vi "Find Repeating Monoclinic GB.vi"(6 "Min Wedge Thickness (A)":dbl=5.0, 8 "Tolerance (A)":dbl=0.5, 9 "Slab Y":dbl=6.0, 10 "Slab X":dbl=6.0, 11 "Supercell Structure":T2={"Structure Name"="CdTe Expanded to Box", "Lattice vector a"=[19.0, 0.0, 0.0], "Lattice vector b"=[0.0, 90.0, 0.0], "Lattice vector c"=[0.0, 0.0, 19.98181818181818], "Atoms Array"=[{"Atom Name"="Cd", "Positions (Direct)"=array501x3[1503 elements], "Positions (Cartesian)"=array501x3[1503 elements]}, {"Atom Name"="Te", "Positions (Direct)"=array504x3[1512 elements], "Positions (Cartesian)"=array504x3[1512 elements]}], "# of atoms"=1005} {"Atoms Array"."Positions (Cartesian)" format="%#_4f"; "Atoms Array"."Positions (Direct)" format="%#_4f"}) -> (1 "Area":dbl, 2 "New Lattice Vector b":dbl[](array[numeric]), 3 "New Lattice Vector a":dbl[](array[numeric]))   [LabVIEW 2010]
panel:
  out "Array 3":dbl[][](array[numeric])
  out "proj":dbl
  out "Possibles from atom 1":dbl[][](array[numeric])
  out "Array 2":dbl[][](array[numeric])
  out "sorted array 2":T1(array[cluster])
  out "All Possible Lattice Vectors":dbl[][](array[numeric]) format="%#_4g"
  out "Slab subset 2":T3(array[cluster])=[{"Atom Name"="Cd", "Positions (Cartesian)"=[[0.0, 4.670554880088597, 0.7469022070093141], [0.0, 0.0, 1.0119047619047619], [0.0, 4.935557434984045, 5.417457087097911], [0.0, 0.2650025548954482, 5.6824596419933595], [0.0, 5.200559989879494, 10.088011967186508], [0.0, 0.5300051097908964, 10.353014522081956], [0.0, 5.465562544774942, 14.758566847275105], [0.0, 0.7950076646863447, 15.023569402170553], [0.0, 5.73056509967039, 19.4291217273637], [0.0, 1.0600102195817929, 19.69412428225915], [3.307892776528626, 2.4677787174920227, 3.2146809245013364], [3.307892776528626, 2.732781272387471, 7.885235804589934], [3.307892776528626, 2.997783827282919, 12.55579068467853], [3.307892776528626, 3.2627863821783674, 17.226345564767126]]}, {"Atom Name"="Te", "Positions (Cartesian)"=[[1.653946388264313, 4.803056157536321, 3.0821796470536116], [1.653946388264313, 0.1325012774477241, 3.3471822019490607], [1.653946388264313, 5.068058712431769, 7.752734527142209], [1.653946388264313, 0.397503832343172, 8.017737082037657], [1.653946388264313, 5.333061267327217, 12.423289407230806], [1.653946388264313, 0.6625063872386205, 12.688291962126254], [1.653946388264313, 5.598063822222666, 17.093844287319403], [1.653946388264313, 0.9275089421340684, 17.358846842214852], [4.96183916479294, 2.3352774400442984, 0.879403484457038], [4.96183916479294, 2.6002799949397466, 5.549958364545636], [4.96183916479294, 2.865282549835195, 10.220513244634233], [4.96183916479294, 3.130285104730643, 14.891068124722828], [4.96183916479294, 3.3952876596260912, 19.561623004811427]]}] {"Positions (Cartesian)" format="%#_4f"}
  out "Supercell without slab":T3(array[cluster])=[{"Atom Name"="Cd", "Positions (Cartesian)"=[0.0, 14.01166464026579, 0.21689709721841766, 0.0, 9.341109760177194, 0.48189965211386543, 0.0, 89.0055452765788, 0.6474110989798403, 0.0, 4.670554880088597, 0.7469022070093141, 0.0, 84.3349903964902, 0.9124136538752889, 0.0, 0.0, 1.0119047619047619, 0.0, 79.6644355164016, 1.1774162087707394, 0.0, 74.993880636313, 1.442418763666188, 0.0, 70.3233257562244, 1.7074213185616385, 0.0, 65.6527708761358, 1.9724238734570871, 0.0, 60.98221599604721, 2.2374264283525305, 0.0, 56.311661115958614, 2.502428983247979, 0.0, 51.64110623587002, 2.7674315381434296, 0.0, 46.97055135578142, 3.0324340930388782, 0.0, 42.29999647569282, 3.297436647934325, 0.0, 37.62944159560422, 3.5624392028297738, 0.0, 32.95888671551563, 3.8274417577252207, 0.0, 28.288331835427034, 4.092444312620669, 0.0, 23.617776955338435, 4.357446867516118, 0.0, 18.947222075249837, 4.622449422411567, 0.0, 14.27666719516124, 4.887451977307014, 0.0, 9.606112315072641, 5.152454532202463, 0.0, 89.27054783147425, 5.317965979068438, 0.0, 4.935557434984045, 5.417457087097911, 0.0, 84.59999295138564, 5.582968533963888, 0.0, 0.2650025548954482, 5.6824596419933595, 0.0, 79.92943807129704, 5.847971088859337, 0.0, 75.25888319120845, 6.1129736437547875, 0.0, 70.58832831111985, 6.377976198650236, 0.0, 65.91777343103126, 6.6429787535456795, 0.0, 61.247218550942655, 6.907981308441128, 0.0, 56.57666367085406, 7.172983863336579, 0.0, 51.906108790765465, 7.437986418232027, 0.0, 47.23555391067687, 7.702988973127474, 0.0, 42.56499903058827, 7.967991528022923, 0.0, 37.89444415049967, 8.23299408291837, 0.0, 33.22388927041108, 8.497996637813818, 0.0, 28.55333439032248, 8.762999192709266, 0.0, 23.882779510233885, 9.028001747604716, 0.0, 19.212224630145286, 9.293004302500165, 0.0, 14.541669750056688, 9.558006857395611, 0.0, 9.87111486996809, 9.82300941229106, 0.0, 89.53555038636969, 9.988520859157038, 0.0, 5.200559989879494, 10.088011967186508, 0.0, 84.86499550628109, 10.253523414052486, 0.0, 0.5300051097908964, 10.353014522081956, 0.0, 80.19444062619249, 10.518525968947937, 0.0, 75.5238857461039, 10.783528523843385, 0.0, 70.85333086601531, 11.04853107873883, 0.0, 66.18277598592671, 11.313533633634277, 0.0, 61.51222110583811, 11.578536188529728, 0.0, 56.841666225749506, 11.843538743425176, 0.0, 52.17111134566091, 12.108541298320624, 0.0, 47.500556465572316, 12.373543853216072, 0.0, 42.83000158548372, 12.63854640811152, 0.0, 38.15944670539512, 12.903548963006967, 0.0, 33.488891825306524, 13.168551517902415, 0.0, 28.81833694521793, 13.433554072797865, 0.0, 24.14778206512933, 13.698556627693314, 0.0, 19.477227185040736, 13.963559182588762, 0.0, 14.806672304952137, 14.22856173748421, 0.0, 10.136117424863539, 14.493564292379657, 0.0, 89.80055294126514, 14.659075739245635, 0.0, 5.465562544774942, 14.758566847275105, 0.0, 85.12999806117654, 14.924078294141086, 0.0, 0.7950076646863447, 15.023569402170553, 0.0, 80.45944318108793, 15.189080849036534, 0.0, 75.78888830099935, 15.454083403931978, 0.0, 71.11833342091076, 15.719085958827426, 0.0, 66.44777854082216, 15.984088513722877, 0.0, 61.777223660733554, 16.249091068618327, 0.0, 57.10666878064496, 16.514093623513773, 0.0, 52.43611390055636, 16.77909617840922, 0.0, 47.76555902046776, 17.04409873330467, 0.0, 43.09500414037917, 17.309101288200118, 0.0, 38.42444926029057, 17.574103843095568, 0.0, 33.75389438020197, 17.839106397991014, 0.0, 29.083339500113375, 18.104108952886463, 0.0, 24.41278462002478, 18.36911150778191, 0.0, 19.74222973993618, 18.63411406267736, 0.0, 15.071674859847585, 18.89911661757281, 0.0, 10.401119979758988, 19.164119172468254, 0.0, 5.73056509967039, 19.4291217273637, 0.0, 85.39500061607198, 19.594633174229685, 0.0, 1.0600102195817929, 19.69412428225915, 0.0, 80.7244457359834, 19.859635729125127, 3.307892776528626, 58.51443727855519, 0.03465026575595598, 3.307892776528626, 53.84388239846659, 0.2996528206514042, 3.307892776528626, 49.173327518377995, 0.5646553755468551, 3.307892776528626, 44.5027726382894, 0.8296579304423033, 3.307892776528626, 39.8322177582008, 1.0946604853377506, 3.307892776528626, 35.161662878112196, 1.3596630402331988, 3.307892776528626, 30.491107998023608, 1.6246655951286462, 3.307892776528626, 25.82055311793501, 1.8896681500240944, 3.307892776528626, 21.14999823784641, 2.1546707049195435, 3.307892776528626, 16.479443357757813, 2.4196732598149917, 3.307892776528626, 11.808888477669216, 2.68467581471044, 3.307892776528626, 7.138333597580619, 2.949678369605888, 3.307892776528626, 86.80276911398222, 3.115189816471863, 3.307892776528626, 2.4677787174920227, 3.2146809245013364, 3.307892776528626, 82.13221423389362, 3.380192371367314, 3.307892776528626, 77.46165935380502, 3.645194926262762, 3.307892776528626, 72.79110447371643, 3.910197481158213, 3.307892776528626, 68.12054959362783, 4.175200036053662, 3.307892776528626, 63.44999471353923, 4.440202590949105, 3.307892776528626, 58.77943983345064, 4.705205145844554, 3.307892776528626, 54.10888495336204, 4.970207700740004, 3.307892776528626, 49.43833007327345, 5.235210255635453, 3.307892776528626, 44.767775193184846, 5.5002128105309, 3.307892776528626, 40.097220313096244, 5.765215365426348, 3.307892776528626, 35.426665433007656, 6.030217920321795, 3.307892776528626, 30.756110552919058, 6.295220475217244, 3.307892776528626, 26.08555567283046, 6.5602230301126925, 3.307892776528626, 21.41500079274186, 6.825225585008141, 3.307892776528626, 16.744445912653262, 7.090228139903589, 3.307892776528626, 12.073891032564665, 7.355230694799037, 3.307892776528626, 7.403336152476069, 7.620233249694485, 3.307892776528626, 87.06777166887767, 7.785744696560463, 3.307892776528626, 2.732781272387471, 7.885235804589934, 3.307892776528626, 82.39721678878907, 8.050747251455912, 3.307892776528626, 77.72666190870048, 8.315749806351363, 3.307892776528626, 73.05610702861188, 8.58075236124681, 3.307892776528626, 68.38555214852329, 8.845754916142255, 3.307892776528626, 63.714997268434686, 9.110757471037703, 3.307892776528626, 59.044442388346084, 9.375760025933154, 3.307892776528626, 54.37388750825748, 9.640762580828602, 3.307892776528626, 49.703332628168894, 9.90576513572405, 3.307892776528626, 45.03277774808029, 10.170767690619497, 3.307892776528626, 40.3622228679917, 10.435770245514945, 3.307892776528626, 35.6916679879031, 10.700772800410393, 3.307892776528626, 31.021113107814504, 10.96577535530584, 3.307892776528626, 26.350558227725905, 11.23077791020129, 3.307892776528626, 21.68000334763731, 11.49578046509674, 3.307892776528626, 17.00944846754871, 11.760783019992187, 3.307892776528626, 12.338893587460113, 12.025785574887635, 3.307892776528626, 7.668338707371516, 12.290788129783083, 3.307892776528626, 87.33277422377311, 12.45629957664906, 3.307892776528626, 2.997783827282919, 12.55579068467853, 3.307892776528626, 82.66221934368451, 12.721302131544512, 3.307892776528626, 77.99166446359591, 12.98630468643996, 3.307892776528626, 73.32110958350734, 13.251307241335404, 3.307892776528626, 68.65055470341873, 13.516309796230852, 3.307892776528626, 63.97999982333013, 13.781312351126303, 3.307892776528626, 59.30944494324153, 14.04631490602175, 3.307892776528626, 54.638890063152935, 14.311317460917198, 3.307892776528626, 49.96833518306434, 14.576320015812646, 3.307892776528626, 45.297780302975745, 14.841322570708094, 3.307892776528626, 40.62722542288715, 15.106325125603542, 3.307892776528626, 35.95667054279855, 15.37132768049899, 3.307892776528626, 31.28611566270995, 15.63633023539444, 3.307892776528626, 26.615560782621355, 15.901332790289889, 3.307892776528626, 21.945005902532756, 16.166335345185335, 3.307892776528626, 17.27445102244416, 16.431337900080784, 3.307892776528626, 12.603896142355563, 16.69634045497623, 3.307892776528626, 7.933341262266964, 16.96134300987168, 3.307892776528626, 87.59777677866856, 17.12685445673766, 3.307892776528626, 3.2627863821783674, 17.226345564767126, 3.307892776528626, 82.92722189857996, 17.391857011633107, 3.307892776528626, 78.25666701849137, 17.656859566528553, 3.307892776528626, 73.58611213840277, 17.921862121424, 3.307892776528626, 68.91555725831418, 18.186864676319452, 3.307892776528626, 64.24500237822558, 18.451867231214898, 3.307892776528626, 59.57444749813698, 18.716869786110347, 3.307892776528626, 54.90389261804839, 18.981872341005793, 3.307892776528626, 50.233337737959786, 19.246874895901243, 3.307892776528626, 45.562782857871184, 19.51187745079669, 3.307892776528626, 40.892227977782596, 19.776880005692142, 6.615785553057252, 14.01166464026579, 0.21689709721841766, 6.615785553057252, 9.341109760177194, 0.48189965211386543, 6.615785553057252, 89.0055452765788, 0.6474110989798403, 6.615785553057252, 4.670554880088597, 0.7469022070093141, 6.615785553057252, 84.3349903964902, 0.9124136538752889, 6.615785553057252, 0.0, 1.0119047619047619, 6.615785553057252, 79.6644355164016, 1.1774162087707394, 6.615785553057252, 74.993880636313, 1.442418763666188, 6.615785553057252, 70.3233257562244, 1.7074213185616385, 6.615785553057252, 65.6527708761358, 1.9724238734570871, 6.615785553057252, 60.98221599604721, 2.2374264283525305, 6.615785553057252, 56.311661115958614, 2.502428983247979, 6.615785553057252, 51.64110623587002, 2.7674315381434296, 6.615785553057252, 46.97055135578142, 3.0324340930388782, 6.615785553057252, 42.29999647569282, 3.297436647934325, 6.615785553057252, 37.62944159560422, 3.5624392028297738, 6.615785553057252, 32.95888671551563, 3.8274417577252207, 6.615785553057252, 28.288331835427034, 4.092444312620669, 6.615785553057252, 23.617776955338435, 4.357446867516118, 6.615785553057252, 18.947222075249837, 4.622449422411567, 6.615785553057252, 14.27666719516124, 4.887451977307014, 6.615785553057252, 9.606112315072641, 5.152454532202463, 6.615785553057252, 89.27054783147425, 5.317965979068438, 6.615785553057252, 4.935557434984045, 5.417457087097911, 6.615785553057252, 84.59999295138564, 5.582968533963888, 6.615785553057252, 0.2650025548954482, 5.6824596419933595, 6.615785553057252, 79.92943807129704, 5.847971088859337, 6.615785553057252, 75.25888319120845, 6.1129736437547875, 6.615785553057252, 70.58832831111985, 6.377976198650236, 6.615785553057252, 65.91777343103126, 6.6429787535456795, 6.615785553057252, 61.247218550942655, 6.907981308441128, 6.615785553057252, 56.57666367085406, 7.172983863336579, 6.615785553057252, 51.906108790765465, 7.437986418232027, 6.615785553057252, 47.23555391067687, 7.702988973127474, 6.615785553057252, 42.56499903058827, 7.967991528022923, 6.615785553057252, 37.89444415049967, 8.23299408291837, 6.615785553057252, 33.22388927041108, 8.497996637813818, 6.615785553057252, 28.55333439032248, 8.762999192709266, 6.615785553057252, 23.882779510233885, 9.028001747604716, 6.615785553057252, 19.212224630145286, 9.293004302500165, 6.615785553057252, 14.541669750056688, 9.558006857395611, 6.615785553057252, 9.87111486996809, 9.82300941229106, 6.615785553057252, 89.53555038636969, 9.988520859157038, 6.615785553057252, 5.200559989879494, 10.088011967186508, 6.615785553057252, 84.86499550628109, 10.253523414052486, 6.615785553057252, 0.5300051097908964, 10.353014522081956, 6.615785553057252, 80.19444062619249, 10.518525968947937, 6.615785553057252, 75.5238857461039, 10.783528523843385, 6.615785553057252, 70.85333086601531, 11.04853107873883, 6.615785553057252, 66.18277598592671, 11.313533633634277, 6.615785553057252, 61.51222110583811, 11.578536188529728, 6.615785553057252, 56.841666225749506, 11.843538743425176, 6.615785553057252, 52.17111134566091, 12.108541298320624, 6.615785553057252, 47.500556465572316, 12.373543853216072, 6.615785553057252, 42.83000158548372, 12.63854640811152, 6.615785553057252, 38.15944670539512, 12.903548963006967, 6.615785553057252, 33.488891825306524, 13.168551517902415, 6.615785553057252, 28.81833694521793, 13.433554072797865, 6.615785553057252, 24.14778206512933, 13.698556627693314, 6.615785553057252, 19.477227185040736, 13.963559182588762, 6.615785553057252, 14.806672304952137, 14.22856173748421, 6.615785553057252, 10.136117424863539, 14.493564292379657, 6.615785553057252, 89.80055294126514, 14.659075739245635, 6.615785553057252, 5.465562544774942, 14.758566847275105, 6.615785553057252, 85.12999806117654, 14.924078294141086, 6.615785553057252, 0.7950076646863447, 15.023569402170553, 6.615785553057252, 80.45944318108793, 15.189080849036534, 6.615785553057252, 75.78888830099935, 15.454083403931978, 6.615785553057252, 71.11833342091076, 15.719085958827426, 6.615785553057252, 66.44777854082216, 15.984088513722877, 6.615785553057252, 61.777223660733554, 16.249091068618327, 6.615785553057252, 57.10666878064496, 16.514093623513773, 6.615785553057252, 52.43611390055636, 16.77909617840922, 6.615785553057252, 47.76555902046776, 17.04409873330467, 6.615785553057252, 43.09500414037917, 17.309101288200118, 6.615785553057252, 38.42444926029057, 17.574103843095568, 6.615785553057252, 33.75389438020197, 17.839106397991014, 6.615785553057252, 29.083339500113375, 18.104108952886463, 6.615785553057252, 24.41278462002478, 18.36911150778191, 6.615785553057252, 19.74222973993618, 18.63411406267736, 6.615785553057252, 15.071674859847585, 18.89911661757281, 6.615785553057252, 10.401119979758988, 19.164119172468254, 6.615785553057252, 5.73056509967039, 19.4291217273637, 6.615785553057252, 85.39500061607198, 19.594633174229685, 6.615785553057252, 1.0600102195817929, 19.69412428225915, 6.615785553057252, 80.7244457359834, 19.859635729125127, 9.92367832958588, 58.51443727855519, 0.03465026575595598, 9.92367832958588, 53.84388239846659, 0.2996528206514042, 9.92367832958588, 49.173327518377995, 0.5646553755468551, 9.92367832958588, 44.5027726382894, 0.8296579304423033, 9.92367832958588, 39.8322177582008, 1.0946604853377506, 9.92367832958588, 35.161662878112196, 1.3596630402331988, 9.92367832958588, 30.491107998023608, 1.6246655951286462, 9.92367832958588, 25.82055311793501, 1.8896681500240944, 9.92367832958588, 21.14999823784641, 2.1546707049195435, 9.92367832958588, 16.479443357757813, 2.4196732598149917, 9.92367832958588, 11.808888477669216, 2.68467581471044, 9.92367832958588, 7.138333597580619, 2.949678369605888, 9.92367832958588, 86.80276911398222, 3.115189816471863, 9.92367832958588, 2.4677787174920227, 3.2146809245013364, 9.92367832958588, 82.13221423389362, 3.380192371367314, 9.92367832958588, 77.46165935380502, 3.645194926262762, 9.92367832958588, 72.79110447371643, 3.910197481158213, 9.92367832958588, 68.12054959362783, 4.175200036053662, 9.92367832958588, 63.44999471353923, 4.440202590949105, 9.92367832958588, 58.77943983345064, 4.705205145844554, 9.92367832958588, 54.10888495336204, 4.970207700740004, 9.92367832958588, 49.43833007327345, 5.235210255635453, 9.92367832958588, 44.767775193184846, 5.5002128105309, 9.92367832958588, 40.097220313096244, 5.765215365426348, 9.92367832958588, 35.426665433007656, 6.030217920321795, 9.92367832958588, 30.756110552919058, 6.295220475217244, 9.92367832958588, 26.08555567283046, 6.5602230301126925, 9.92367832958588, 21.41500079274186, 6.825225585008141, 9.92367832958588, 16.744445912653262, 7.090228139903589, 9.92367832958588, 12.073891032564665, 7.355230694799037, 9.92367832958588, 7.403336152476069, 7.620233249694485, 9.92367832958588, 87.06777166887767, 7.785744696560463, 9.92367832958588, 2.732781272387471, 7.885235804589934, 9.92367832958588, 82.39721678878907, 8.050747251455912, 9.92367832958588, 77.72666190870048, 8.315749806351363, 9.92367832958588, 73.05610702861188, 8.58075236124681, 9.92367832958588, 68.38555214852329, 8.845754916142255, 9.92367832958588, 63.714997268434686, 9.110757471037703, 9.92367832958588, 59.044442388346084, 9.375760025933154, 9.92367832958588, 54.37388750825748, 9.640762580828602, 9.92367832958588, 49.703332628168894, 9.90576513572405, 9.92367832958588, 45.03277774808029, 10.170767690619497, 9.92367832958588, 40.3622228679917, 10.435770245514945, 9.92367832958588, 35.6916679879031, 10.700772800410393, 9.92367832958588, 31.021113107814504, 10.96577535530584, 9.92367832958588, 26.350558227725905, 11.23077791020129, 9.92367832958588, 21.68000334763731, 11.49578046509674, 9.92367832958588, 17.00944846754871, 11.760783019992187, 9.92367832958588, 12.338893587460113, 12.025785574887635, 9.92367832958588, 7.668338707371516, 12.290788129783083, 9.92367832958588, 87.33277422377311, 12.45629957664906, 9.92367832958588, 2.997783827282919, 12.55579068467853, 9.92367832958588, 82.66221934368451, 12.721302131544512, 9.92367832958588, 77.99166446359591, 12.98630468643996, 9.92367832958588, 73.32110958350734, 13.251307241335404, 9.92367832958588, 68.65055470341873, 13.516309796230852, 9.92367832958588, 63.97999982333013, 13.781312351126303, 9.92367832958588, 59.30944494324153, 14.04631490602175, 9.92367832958588, 54.638890063152935, 14.311317460917198, 9.92367832958588, 49.96833518306434, 14.576320015812646, 9.92367832958588, 45.297780302975745, 14.841322570708094, 9.92367832958588, 40.62722542288715, 15.106325125603542, 9.92367832958588, 35.95667054279855, 15.37132768049899, 9.92367832958588, 31.28611566270995, 15.63633023539444, 9.92367832958588, 26.615560782621355, 15.901332790289889, 9.92367832958588, 21.945005902532756, 16.166335345185335, 9.92367832958588, 17.27445102244416, 16.431337900080784, 9.92367832958588, 12.603896142355563, 16.69634045497623, 9.92367832958588, 7.933341262266964, 16.96134300987168, 9.92367832958588, 87.59777677866856, 17.12685445673766, 9.92367832958588, 3.2627863821783674, 17.226345564767126, 9.92367832958588, 82.92722189857996, 17.391857011633107, 9.92367832958588, 78.25666701849137, 17.656859566528553, 9.92367832958588, 73.58611213840277, 17.921862121424, 9.92367832958588, 68.91555725831418, 18.186864676319452, 9.92367832958588, 64.24500237822558, 18.451867231214898, 9.92367832958588, 59.57444749813698, 18.716869786110347, 9.92367832958588, 54.90389261804839, 18.981872341005793, 9.92367832958588, 50.233337737959786, 19.246874895901243, 9.92367832958588, 45.562782857871184, 19.51187745079669, 9.92367832958588, 40.892227977782596, 19.776880005692142, 13.231571106114504, 14.01166464026579, 0.21689709721841766, 13.231571106114504, 9.341109760177194, 0.48189965211386543, 13.231571106114504, 89.0055452765788, 0.6474110989798403, 13.231571106114504, 4.670554880088597, 0.7469022070093141, 13.231571106114504, 84.3349903964902, 0.9124136538752889, 13.231571106114504, 0.0, 1.0119047619047619, 13.231571106114504, 79.6644355164016, 1.1774162087707394, 13.231571106114504, 74.993880636313, 1.442418763666188, 13.231571106114504, 70.3233257562244, 1.7074213185616385, 13.231571106114504, 65.6527708761358, 1.9724238734570871, 13.231571106114504, 60.98221599604721, 2.2374264283525305, 13.231571106114504, 56.311661115958614, 2.502428983247979, 13.231571106114504, 51.64110623587002, 2.7674315381434296, 13.231571106114504, 46.97055135578142, 3.0324340930388782, 13.231571106114504, 42.29999647569282, 3.297436647934325, 13.231571106114504, 37.62944159560422, 3.5624392028297738, 13.231571106114504, 32.95888671551563, 3.8274417577252207, 13.231571106114504, 28.288331835427034, 4.092444312620669, 13.231571106114504, 23.617776955338435, 4.357446867516118, 13.231571106114504, 18.947222075249837, 4.622449422411567, 13.231571106114504, 14.27666719516124, 4.887451977307014, 13.231571106114504, 9.606112315072641, 5.152454532202463, 13.231571106114504, 89.27054783147425, 5.317965979068438, 13.231571106114504, 4.935557434984045, 5.417457087097911, 13.231571106114504, 84.59999295138564, 5.582968533963888, 13.231571106114504, 0.2650025548954482, 5.6824596419933595, 13.231571106114504, 79.92943807129704, 5.847971088859337, 13.231571106114504, 75.25888319120845, 6.1129736437547875, 13.231571106114504, 70.58832831111985, 6.377976198650236, 13.231571106114504, 65.91777343103126, 6.6429787535456795, 13.231571106114504, 61.247218550942655, 6.907981308441128, 13.231571106114504, 56.57666367085406, 7.172983863336579, 13.231571106114504, 51.906108790765465, 7.437986418232027, 13.231571106114504, 47.23555391067687, 7.702988973127474, 13.231571106114504, 42.56499903058827, 7.967991528022923, 13.231571106114504, 37.89444415049967, 8.23299408291837, 13.231571106114504, 33.22388927041108, 8.497996637813818, 13.231571106114504, 28.55333439032248, 8.762999192709266, 13.231571106114504, 23.882779510233885, 9.028001747604716, 13.231571106114504, 19.212224630145286, 9.293004302500165, 13.231571106114504, 14.541669750056688, 9.558006857395611, 13.231571106114504, 9.87111486996809, 9.82300941229106, 13.231571106114504, 89.53555038636969, 9.988520859157038, 13.231571106114504, 5.200559989879494, 10.088011967186508, 13.231571106114504, 84.86499550628109, 10.253523414052486, 13.231571106114504, 0.5300051097908964, 10.353014522081956, 13.231571106114504, 80.19444062619249, 10.518525968947937, 13.231571106114504, 75.5238857461039, 10.783528523843385, 13.231571106114504, 70.85333086601531, 11.04853107873883, 13.231571106114504, 66.18277598592671, 11.313533633634277, 13.231571106114504, 61.51222110583811, 11.578536188529728, 13.231571106114504, 56.841666225749506, 11.843538743425176, 13.231571106114504, 52.17111134566091, 12.108541298320624, 13.231571106114504, 47.500556465572316, 12.373543853216072, 13.231571106114504, 42.83000158548372, 12.63854640811152, 13.231571106114504, 38.15944670539512, 12.903548963006967, 13.231571106114504, 33.488891825306524, 13.168551517902415, 13.231571106114504, 28.81833694521793, 13.433554072797865, 13.231571106114504, 24.14778206512933, 13.698556627693314, 13.231571106114504, 19.477227185040736, 13.963559182588762, 13.231571106114504, 14.806672304952137, 14.22856173748421, 13.231571106114504, 10.136117424863539, 14.493564292379657, 13.231571106114504, 89.80055294126514, 14.659075739245635, 13.231571106114504, 5.465562544774942, 14.758566847275105, 13.231571106114504, 85.12999806117654, 14.924078294141086, 13.231571106114504, 0.7950076646863447, 15.023569402170553, 13.231571106114504, 80.45944318108793, 15.189080849036534, 13.231571106114504, 75.78888830099935, 15.454083403931978, 13.231571106114504, 71.11833342091076, 15.719085958827426, 13.231571106114504, 66.44777854082216, 15.984088513722877, 13.231571106114504, 61.777223660733554, 16.249091068618327, 13.231571106114504, 57.10666878064496, 16.514093623513773, 13.231571106114504, 52.43611390055636, 16.77909617840922, 13.231571106114504, 47.76555902046776, 17.04409873330467, 13.231571106114504, 43.09500414037917, 17.309101288200118, 13.231571106114504, 38.42444926029057, 17.574103843095568, 13.231571106114504, 33.75389438020197, 17.839106397991014, 13.231571106114504, 29.083339500113375, 18.104108952886463, 13.231571106114504, 24.41278462002478, 18.36911150778191, 13.231571106114504, 19.74222973993618, 18.63411406267736, 13.231571106114504, 15.071674859847585, 18.89911661757281, 13.231571106114504, 10.401119979758988, 19.164119172468254, 13.231571106114504, 5.73056509967039, 19.4291217273637, 13.231571106114504, 85.39500061607198, 19.594633174229685, 13.231571106114504, 1.0600102195817929, 19.69412428225915, 13.231571106114504, 80.7244457359834, 19.859635729125127, 16.53946388264313, 58.51443727855519, 0.03465026575595598, 16.53946388264313, 53.84388239846659, 0.2996528206514042, 16.53946388264313, 49.173327518377995, 0.5646553755468551, 16.53946388264313, 44.5027726382894, 0.8296579304423033, 16.53946388264313, 39.8322177582008, 1.0946604853377506, 16.53946388264313, 35.161662878112196, 1.3596630402331988, 16.53946388264313, 30.491107998023608, 1.6246655951286462, 16.53946388264313, 25.82055311793501, 1.8896681500240944, 16.53946388264313, 21.14999823784641, 2.1546707049195435, 16.53946388264313, 16.479443357757813, 2.4196732598149917, 16.53946388264313, 11.808888477669216, 2.68467581471044, 16.53946388264313, 7.138333597580619, 2.949678369605888, 16.53946388264313, 86.80276911398222, 3.115189816471863, 16.53946388264313, 2.4677787174920227, 3.2146809245013364, 16.53946388264313, 82.13221423389362, 3.380192371367314, 16.53946388264313, 77.46165935380502, 3.645194926262762, 16.53946388264313, 72.79110447371643, 3.910197481158213, 16.53946388264313, 68.12054959362783, 4.175200036053662, 16.53946388264313, 63.44999471353923, 4.440202590949105, 16.53946388264313, 58.77943983345064, 4.705205145844554, 16.53946388264313, 54.10888495336204, 4.970207700740004, 16.53946388264313, 49.43833007327345, 5.235210255635453, 16.53946388264313, 44.767775193184846, 5.5002128105309, 16.53946388264313, 40.097220313096244, 5.765215365426348, 16.53946388264313, 35.426665433007656, 6.030217920321795, 16.53946388264313, 30.756110552919058, 6.295220475217244, 16.53946388264313, 26.08555567283046, 6.5602230301126925, 16.53946388264313, 21.41500079274186, 6.825225585008141, 16.53946388264313, 16.744445912653262, 7.090228139903589, 16.53946388264313, 12.073891032564665, 7.355230694799037, 16.53946388264313, 7.403336152476069, 7.620233249694485, 16.53946388264313, 87.06777166887767, 7.785744696560463, 16.53946388264313, 2.732781272387471, 7.885235804589934, 16.53946388264313, 82.39721678878907, 8.050747251455912, 16.53946388264313, 77.72666190870048, 8.315749806351363, 16.53946388264313, 73.05610702861188, 8.58075236124681, 16.53946388264313, 68.38555214852329, 8.845754916142255, 16.53946388264313, 63.714997268434686, 9.110757471037703, 16.53946388264313, 59.044442388346084, 9.375760025933154, 16.53946388264313, 54.37388750825748, 9.640762580828602, 16.53946388264313, 49.703332628168894, 9.90576513572405, 16.53946388264313, 45.03277774808029, 10.170767690619497, 16.53946388264313, 40.3622228679917, 10.435770245514945, 16.53946388264313, 35.6916679879031, 10.700772800410393, 16.53946388264313, 31.021113107814504, 10.96577535530584, 16.53946388264313, 26.350558227725905, 11.23077791020129, 16.53946388264313, 21.68000334763731, 11.49578046509674, 16.53946388264313, 17.00944846754871, 11.760783019992187, 16.53946388264313, 12.338893587460113, 12.025785574887635, 16.53946388264313, 7.668338707371516, 12.290788129783083, 16.53946388264313, 87.33277422377311, 12.45629957664906, 16.53946388264313, 2.997783827282919, 12.55579068467853, 16.53946388264313, 82.66221934368451, 12.721302131544512, 16.53946388264313, 77.99166446359591, 12.98630468643996, 16.53946388264313, 73.32110958350734, 13.251307241335404, 16.53946388264313, 68.65055470341873, 13.516309796230852, 16.53946388264313, 63.97999982333013, 13.781312351126303, 16.53946388264313, 59.30944494324153, 14.04631490602175, 16.53946388264313, 54.638890063152935, 14.311317460917198, 16.53946388264313, 49.96833518306434, 14.576320015812646, 16.53946388264313, 45.297780302975745, 14.841322570708094, 16.53946388264313, 40.62722542288715, 15.106325125603542, 16.53946388264313, 35.95667054279855, 15.37132768049899, 16.53946388264313, 31.28611566270995, 15.63633023539444, 16.53946388264313, 26.615560782621355, 15.901332790289889, 16.53946388264313, 21.945005902532756, 16.166335345185335, 16.53946388264313, 17.27445102244416, 16.431337900080784, 16.53946388264313, 12.603896142355563, 16.69634045497623, 16.53946388264313, 7.933341262266964, 16.96134300987168, 16.53946388264313, 87.59777677866856, 17.12685445673766, 16.53946388264313, 3.2627863821783674, 17.226345564767126, 16.53946388264313, 82.92722189857996, 17.391857011633107, 16.53946388264313, 78.25666701849137, 17.656859566528553, 16.53946388264313, 73.58611213840277, 17.921862121424, 16.53946388264313, 68.91555725831418, 18.186864676319452, 16.53946388264313, 64.24500237822558, 18.451867231214898, 16.53946388264313, 59.57444749813698, 18.716869786110347, 16.53946388264313, 54.90389261804839, 18.981872341005793, 16.53946388264313, 50.233337737959786, 19.246874895901243, 16.53946388264313, 45.562782857871184, 19.51187745079669, 16.53946388264313, 40.892227977782596, 19.776880005692142]}, ...(2 in all)] {"Positions (Cartesian)" format="%#_4f"}
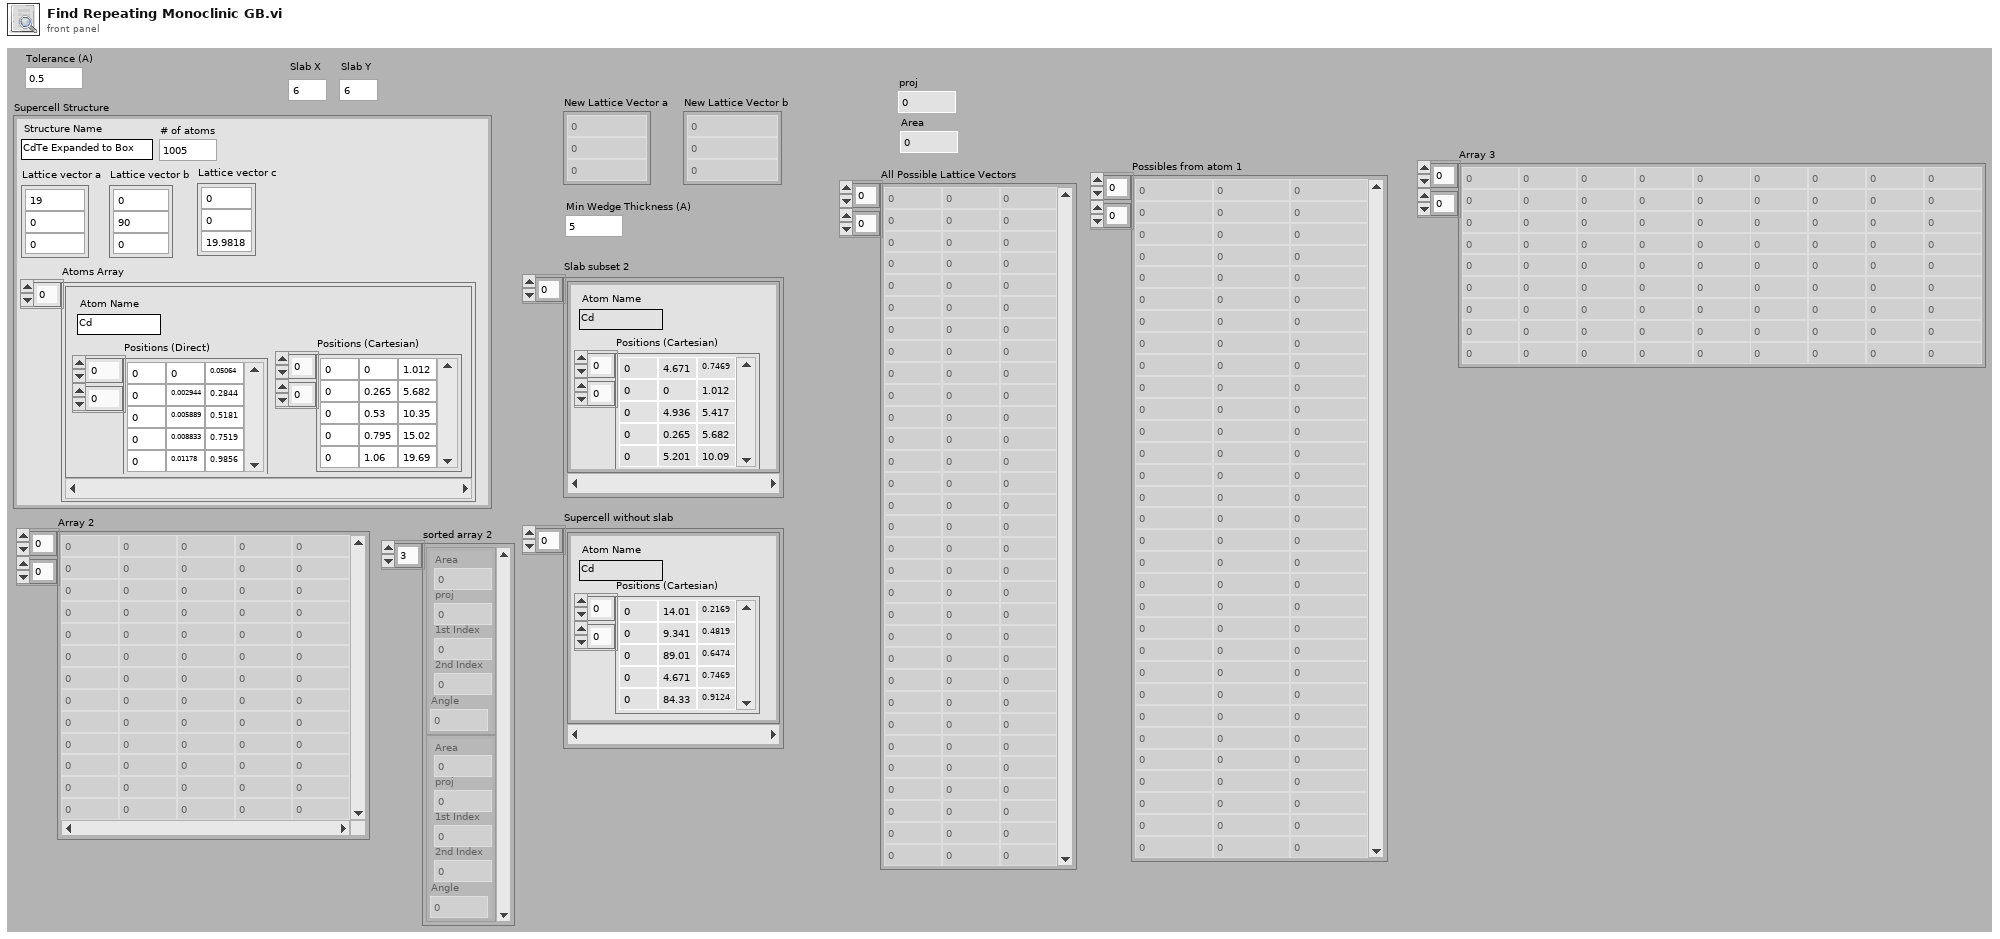
[diagram p1: front panel]
types:
  T1 = cluster{"Area":dbl, "proj":dbl, "1st Index":i32, "2nd Index":i32, "Angle":dbl}[]
  T2 = cluster{"Structure Name":string, "Lattice vector a":dbl[], "Lattice vector b":dbl[], "Lattice vector c":dbl[], "Atoms Array":cluster{"Atom Name":string, "Positions (Direct)":dbl[][], "Positions (Cartesian)":dbl[][]}[], "# of atoms":i32}
  T3 = cluster{"Atom Name":string, "Positions (Cartesian)":dbl[][]}[]
  T4 = cluster{"Atom Name":string, "Positions (Direct)":dbl[][], "Positions (Cartesian)":dbl[][]}[]
  T5 = cluster{dbl, dbl, i32, i32, "Angle (Degrees)":dbl}
  T6 = cluster{"Area":dbl, "proj":dbl, "1st Index":i32, "2nd Index":i32, "Angle (Degrees)":dbl}[]
  T7 = cluster{"Area":dbl, "proj":dbl, "1st Index":i32, "2nd Index":i32, "Angle":dbl}
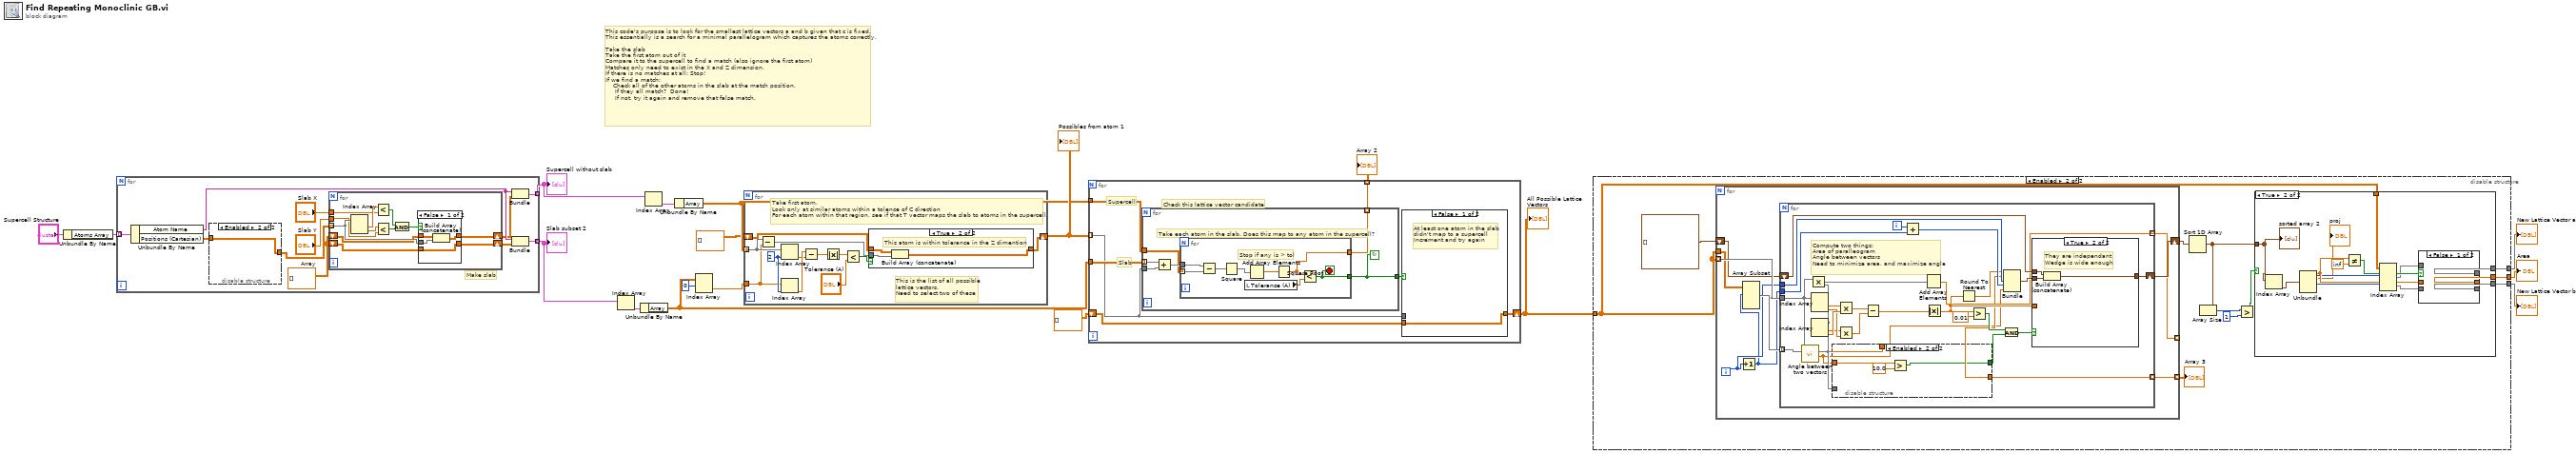
[diagram p0: block diagram]
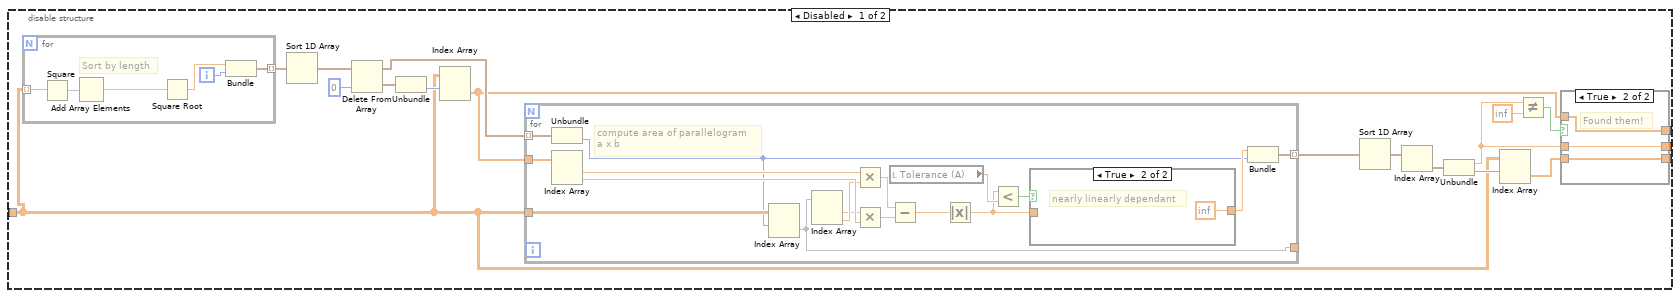
[diagram p2: hidden frame]
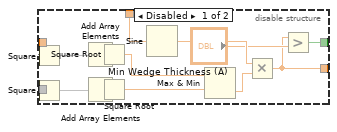
[diagram p7: hidden frame]
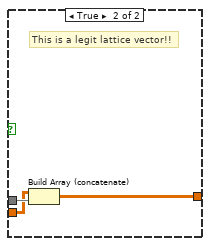
[diagram p9: hidden frame]
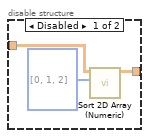
[diagram p11: hidden frame]
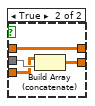
[diagram p12: hidden frame]
diagram:
  # "This code's purpose is to look for the smallest lattice vectors a and b given that c is fixed.\nThis essentially is a search for a minimal parallelogram which captures the atoms correctly.\n\nTake the slab\nTake the first atom out of it\nCompare it to the supercell to find a match (also ignore the first atom)\nMatches only need to exist in the X and Z dimension.\nIf there is no matches at all: Stop!\nIf we find a match: \n    Check all of the other atoms in the slab at the match position.\n     If they all match?  Done!\n     If not, try it again and remove that false match."
  n1 = Unbundle By Name("Supercell Structure") -> ("Atoms Array"=w15:T4)
  n2 = for {
    tunnel: w15 -> [w29] mode=indexing
    tunnel: [w26] -> w13 mode=indexing
    tunnel: [w21] -> w12 mode=indexing
    w20 = dbl[][] []  # Array
    # "Make slab"
    n3 = Unbundle By Name(w29) -> ("Atom Name"=w22:string, "Positions (Cartesian)"=w24:dbl[][])
    n4 = disable-structure shown="Enabled" {
      disable-tunnel: w24 -> [w31 w33]
      disable-tunnel: [w30 w33] -> w23
      frame Disabled {
        n5 = call "Sort 2D Array (Numeric).vi"("Sort by Cols"=i32[] [0, 1, 2], "Input Array"=w31) -> ("Output Array"=w30:dbl[][])  [unwired: 9 in]
      }
      frame Enabled {
      }
    }
    n6 = for {
      tunnel: w23 -> [w43] mode=indexing
      shift-right: [w45] -> w25
      shift-left: w20 -> [w44]
      tunnel: "Slab X" -> [w41]
      tunnel: "Slab Y" -> [w39]
      shift-right: [w35] -> w19
      shift-left: w20 -> [w34]
      n7 = Index Array(array=w43) -> (element #1=w42:dbl, element #2=w40:dbl)  [unwired: 2 in]
      n8 = Less?(x=w42, y=w41) -> (x < y?=w38:bool)
      n9 = Less?(x=w40, y=w39) -> (x < y?=w37:bool)
      n10 = And(x=w38, y=w37) -> (x .and. y?=w36:bool)
      n11 = case shown="False" w36 {
        tunnel: w43 -> [w48 w53]
        tunnel: [w49 w52] -> w45
        tunnel: w44 -> [w49 w51]
        tunnel: [w47 w50] -> w35
        tunnel: w34 -> [w46 w50]
        frame False {
          n12 = Build Array (concatenate)(w46, w48) -> (w47:dbl[][])
        }
        frame True {
          n13 = Build Array (concatenate)(w51, w53) -> (w52:dbl[][])
        }
      }
    }
    n14 = Bundle("Atom Name"=w22, "Array"=w19) -> (w21:cluster{"Atom Name":string, "Array":dbl[][]})  [unwired: 1 in]
    n15 = Bundle("Atom Name"=w22, "Array"=w25) -> (w26:cluster{"Atom Name":string, "Array":dbl[][]})  [unwired: 1 in]
  }
  "Supercell without slab" <- w12
  "Slab subset 2" <- w13
  n16 = Index Array(array=w13) -> (element=w17:cluster{"Atom Name":string, "Array":dbl[][]})  [unwired: 1 in]
  n17 = Unbundle By Name(w17) -> ("Array"=w3:dbl[][])
  n18 = Index Array(array=w12) -> (element=w18:cluster{"Atom Name":string, "Array":dbl[][]})  [unwired: 1 in]
  n19 = Unbundle By Name(w18) -> ("Array"=w4:dbl[][])
  n20 = Index Array(array=w3, index (row)=0) -> (element=w11:dbl[])  [unwired: 1 in]
  n21 = for {
    tunnel: w11 -> [w56]
    tunnel: w4 -> [w57] mode=indexing
    shift-right: [w59] -> w10
    shift-left: dbl[][] [] -> [w58]
    w65 = 2 ("index")
    # "Take first atom.\nLook only at similar atoms within a tolence of C direction\nFor each atom within that region, see if that T vector maps the slab to atoms in the supercell."
    # "This is the list of all possible\nlattice vectors.\nNeed to select two of these"
    n22 = Subtract(x=w57, y=w56) -> (x-y=w55:dbl[])
    n23 = Index Array(array=w57, index=w65) -> (element=w63:dbl)
    n24 = Index Array(array=w56, index=w65) -> (element=w64:dbl)
    n25 = Subtract(x=w64, y=w63) -> (x-y=w62:dbl)
    n26 = Absolute Value(x=w62) -> (abs(x)=w61:dbl)
    n27 = Less?(x=w61, y="Tolerance (A)") -> (x < y?=w60:bool)
    n28 = case shown="True" w60 {
      tunnel: w55 -> [_ w69]
      tunnel: [w66 w68] -> w59
      tunnel: w58 -> [w66 w67]
      frame False {
      }
      frame True {
        # "This atom is within tolerance in the Z dimention"
        n29 = Build Array (concatenate)(w67, w69) -> (w68:dbl[][])
      }
    }
  }
  "Possibles from atom 1" <- w10
  n30 = for {
    tunnel: w10 -> [w73] mode=indexing
    tunnel: w3 -> [w76]
    tunnel: w4 -> [w75]
    shift-right: [w72] -> w5
    shift-left: dbl[][] [] -> [w71]
    tunnel: [w70] -> w1 mode=indexing
    # "Supercell"
    # "Slab"
    # "Check this lattice vector candidate"
    n31 = for {
      tunnel: w76 -> [w86] mode=indexing
      tunnel: w73 -> [w85]
      tunnel: w75 -> [w83]
      tunnel: [w82] -> w74
      tunnel: [w81] -> w70 mode=indexing
      stop <- w82 continue-if-true
      # "Take each atom in the slab. Does this map to any atom in the supercell?"
      n32 = Add(x=w86, y=w85) -> (x+y=w84:dbl[])
      n33 = for {
        tunnel: w84 -> [w94]
        tunnel: w83 -> [w93] mode=indexing
        tunnel: [w88] -> w82
        tunnel: [w87] -> w81
        stop <- w88 stop-if-true
        # "Stop if any is > tol"
        n34 = Subtract(x=w94, y=w93) -> (x-y=w92:dbl[])
        n35 = Square(x=w92) -> (x^2=w91:dbl[])
        n36 = local read "Tolerance (A)"() -> (w89:dbl)
        n37 = Add Array Elements(numeric array=w91) -> (sum=w90:dbl)
        n38 = Square Root(x=w90) -> (sqrt(x)=w87:dbl)
        n39 = Less?(x=w87, y=w89) -> (x < y?=w88:bool)
      }
    }
    n40 = case shown="False" w74 {
      tunnel: w73 -> [_ w80]
      tunnel: [w77 w79] -> w72
      tunnel: w71 -> [w77 w78]
      frame False {
        # "At least one atom in the slab\ndidn't map to a supercell\nIncrement and try again"
      }
      frame True {
        # "This is a legit lattice vector!!"
        n41 = Build Array (concatenate)(w78, w80) -> (w79:dbl[][])
      }
    }
  }
  "All Possible Lattice Vectors" <- w5
  "Array 2" <- w1
  n42 = disable-structure shown="Enabled" {
    disable-tunnel: [w106 w149] -> w8
    disable-tunnel: [w105 w148] -> w7
    disable-tunnel: [w98 w147] -> w6
    disable-tunnel: w5 -> [w95 w150]
    frame Disabled {
      n43 = for {
        tunnel: w95 -> [w136] mode=indexing
        tunnel: [w133] -> w113 mode=indexing
        i -> [w135]
        # "Sort by length"
        n44 = Square(x=w136) -> (x^2=w137:dbl[])
        n45 = Add Array Elements(numeric array=w137) -> (sum=w138:dbl)
        n46 = Square Root(x=w138) -> (sqrt(x)=w134:dbl)
        n47 = Bundle(w134, w135) -> (w133:cluster{dbl, i32})  [unwired: 1 in]
      }
      n48 = Sort 1D Array(array=w113) -> (sorted array=w111:cluster{dbl, i32}[])
      n49 = Delete From Array(array=w111, index=0) -> (deleted portion=w109:cluster{dbl, i32}, array with subset deleted=w108:cluster{dbl, i32}[])  [unwired: 1 in]
      n50 = Unbundle(w109) -> (w112:i32)  [unwired: 1 out]
      n51 = Index Array(array=w95, index (row)=w112) -> (element=w107:dbl[])  [unwired: 1 in]
      n52 = for {
        tunnel: w107 -> [w128]
        tunnel: w108 -> [w130] mode=indexing
        tunnel: w95 -> [w129]
        tunnel: [w123] -> _
        tunnel: [w114] -> w104 mode=indexing
        # "compute area of parallelogram\na x b"
        n53 = Unbundle(w130) -> (w115:i32)  [unwired: 1 out]
        n54 = Index Array(array=w128) -> (element #1=w127:dbl, element #2=w126:dbl)  [unwired: 2 in]
        n55 = Index Array(array=w129, index (row)=w115) -> (element=w123:dbl[])  [unwired: 1 in]
        n56 = Index Array(array=w123) -> (element #1=w124:dbl, element #2=w125:dbl)  [unwired: 2 in]
        n57 = Multiply(x=w127, y=w125) -> (x*y=w122:dbl)
        n58 = Multiply(x=w124, y=w126) -> (x*y=w121:dbl)
        n59 = local read "Tolerance (A)"() -> (w119:dbl)
        n60 = Subtract(x=w122, y=w121) -> (x-y=w120:dbl)
        n61 = Absolute Value(x=w120) -> (abs(x)=w117:dbl)
        n62 = Less?(x=w117, y=w119) -> (x < y?=w118:bool)
        n63 = case shown="True" w118 {
          tunnel: w117 -> [w131 _]
          tunnel: [w131 inf] -> w116
          frame False {
            # "Independant\nwith area given by..."
          }
          frame True {
            # "nearly linearly dependant"
          }
        }
        n64 = Bundle(w116, w115) -> (w114:cluster{dbl, i32})  [unwired: 1 in]
      }
      n65 = Sort 1D Array(array=w104) -> (sorted array=w96:cluster{dbl, i32}[])
      n66 = Index Array(array=w96) -> (element=w103:cluster{dbl, i32})  [unwired: 1 in]
      n67 = Unbundle(w103) -> (w97:dbl, w102:i32)
      n68 = Index Array(array=w95, index (row)=w102) -> (element=w101:dbl[])  [unwired: 1 in]
      n69 = Not Equal?(x=w97, y=inf) -> (x != y?=w99:bool)
      n70 = case shown="True" w99 {
        tunnel: w107 -> [_ w141]
        tunnel: w101 -> [_ w140]
        tunnel: [_ w141] -> w106
        tunnel: [_ w140] -> w105
        tunnel: [_ w139] -> w98
        tunnel: w97 -> [_ w139]
        frame False {
        }
        frame True {
          # "Found them!"
        }
      }
    }
    frame Enabled {
      n71 = for {
        tunnel: w150 -> [w178] mode=indexing
        tunnel: w150 -> [w177]
        shift-right: [w173] -> w151
        shift-left: T1 [] -> [w174]
        tunnel: [w171] -> _ mode=indexing
        tunnel: [w170] -> w142 mode=indexing
        i -> [w175]
        n72 = Increment(x=w175) -> (x+1=w172:i32)
        n73 = Array Subset(array=w177, index (row)=w172) -> (w176:dbl[][])  [unwired: 3 in]
        n74 = for {
          tunnel: w178 -> [w187]
          tunnel: w176 -> [w186] mode=indexing
          tunnel: w175 -> [w197]
          shift-right: [w191] -> w173
          shift-left: w174 -> [w192]
          tunnel: w172 -> [w195]
          tunnel: [w185] -> w171 mode=indexing
          tunnel: [w181] -> w170 mode=indexing
          i -> [w196]
          # "Compute two things:\nArea of paralleogram\nAngle between vectors\nNeed to minimize area, and maximize angle"
          n75 = call "Angle between two vectors.vi"("Vector 2"=w186, "Vector 1"=w187) -> ("Angle (Degrees)"=w179:dbl, "Angle (Radians)"=w183:dbl)  [unwired: 7 in, 1 out]
          n76 = Multiply(x=w187, y=w186) -> (x*y=w198:dbl[])
          n77 = Index Array(array=w187) -> (element #1=w205:dbl, element #2=w203:dbl)  [unwired: 2 in]
          n78 = Index Array(array=w186) -> (element #1=w202:dbl, element #2=w204:dbl)  [unwired: 2 in]
          n79 = disable-structure shown="Enabled" {
            disable-tunnel: w186 -> [w217 _]
            disable-tunnel: w183 -> [w210 _]
            disable-tunnel: [w207 _] -> w181
            disable-tunnel: [w206 w219] -> w180
            disable-tunnel: w179 -> [_ w221]
            frame Disabled {
              n80 = Square(x=w217) -> (x^2=w218:dbl[])
              n81 = Square(x=w217) -> (x^2=w216:dbl[])
              n82 = Add Array Elements(numeric array=w218) -> (sum=w215:dbl)
              n83 = Add Array Elements(numeric array=w216) -> (sum=w214:dbl)
              n84 = Square Root(x=w215) -> (sqrt(x)=w213:dbl)
              n85 = Square Root(x=w214) -> (sqrt(x)=w212:dbl)
              n86 = Sine(x=w210) -> (sin(x)=w209:dbl)
              n87 = Max & Min(x=w213, y=w212) -> (min(x,y)=w211:dbl)  [unwired: 1 out]
              n88 = Multiply(x=w209, y=w211) -> (x*y=w207:dbl)
              n89 = Greater?(x=w207, y="Min Wedge Thickness (A)") -> (0:w206:bool)
            }
            frame Enabled {
              n90 = Greater?(x=w221, y=10.0) -> (0:w219:bool)
            }
          }
          n91 = Multiply(x=w205, y=w204) -> (x*y=w201:dbl)
          n92 = Multiply(x=w202, y=w203) -> (x*y=w200:dbl)
          n93 = Subtract(x=w201, y=w200) -> (x-y=w199:dbl)
          n94 = Add(x=w196, y=w195) -> (x+y=w194:i32)
          n95 = Add Array Elements(numeric array=w198) -> (sum=w185:dbl)
          n96 = Absolute Value(x=w199) -> (abs(x)=w190:dbl)
          n97 = Round To Nearest(number=w190) -> (nearest integer value=w189:dbl)
          n98 = Greater?(x=w190, y=0.01) -> (0:w184:bool)
          n99 = And(x=w184, y=w180) -> (x .and. y?=w182:bool)
          n100 = Bundle(w189, w181, w197, w194, "Angle (Degrees)"=w179) -> (w188:T5)  [unwired: 1 in]
          n101 = case shown="True" w182 {
            tunnel: w190 -> [_ _]
            tunnel: w192 -> [w222 w225]
            tunnel: [w222 w223] -> w191
            tunnel: w188 -> [_ w224]
            frame False {
              # "nearly linearly dependant"
            }
            frame True {
              # "They are independant\nWedge is wide enough"
              n102 = Build Array (concatenate)(w225, w224) -> (w223:T6)
            }
          }
        }
      }
      "Array 3" <- w142
      n103 = Sort 1D Array(array=w151) -> (sorted array=w146:T1)
      n104 = Array Size(array=w146) -> (size(s)=w145:i32)
      n105 = Greater?(x=w145, y=1) -> (0:w143:bool)
      n106 = case shown="True" w143 {
        tunnel: w150 -> [_ w162]
        tunnel: [_ w158] -> w149
        tunnel: [_ w156] -> w148
        tunnel: [_ w155] -> w147
        tunnel: w146 -> [_ w153]
        frame False {
        }
        frame True {
          n107 = Index Array(array=w153) -> (element=w163:T7)  [unwired: 1 in]
          n108 = Unbundle(w163) -> ("Area"=w164:dbl, "proj"=→"proj":dbl, "1st Index"=w161:i32, "2nd Index"=w160:i32)  [unwired: 1 out]
          n109 = Not Equal?(x=w164, y=inf) -> (x != y?=w165:bool)
          n110 = Index Array(array=w162, index (row) #1=w161, index (row) #2=w160) -> (element #1=w159:dbl[], element #2=w157:dbl[])  [unwired: 2 in]
          n111 = case shown="False" w165 {
            tunnel: w159 -> [_ w169]
            tunnel: w157 -> [_ w168]
            tunnel: [_ w169] -> w158
            tunnel: [_ w168] -> w156
            tunnel: [_ w167] -> w155
            tunnel: w164 -> [_ w167]
            frame False {
            }
            frame True {
              # "Found them!"
            }
          }
          "sorted array 2" <- w153
        }
      }
    }
  }
  "New Lattice Vector a" <- w8
  "New Lattice Vector b" <- w7
  "Area" <- w6
